vi "Get DIP State.vi"(8 "error in (no error)":errorcluster) -> (0 "error out":errorcluster, 3 "DIP State":u32)   [LabVIEW 2016]
uses:
  Refname/Sensors.ctl
  Refname/Refname to String (Sensors).vi
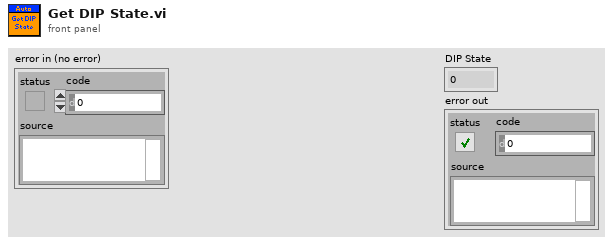
[diagram p1: front panel]
types:
  T1 = typedef "Sensors.ctl" = enum16{"DIP 1", "DIP 2", "DIP 3", "DIP 4", "IMU", "HuskieBoard"}
  T2 = typedef "WPI_SwitchDevRef.ctl" = cluster{"DevStatus":errorcluster, "DIO Channel":T3, "CntIndex":T4, "Normally Closed":bool}
  T3 = typedef "FPGA_DIOChannel.ctl" = enum8{"DIO 0", "DIO 1", "DIO 2", "DIO 3", "DIO 4", "DIO 5", "DIO 6", "DIO 7", "DIO 8", "DIO 9", "DIO MXP 0", "DIO MXP 1", "DIO MXP 2", "DIO MXP 3", "DIO MXP 4", "DIO MXP 5", "DIO MXP 6", "DIO MXP 7", "DIO MXP 8", "DIO MXP 9", "DIO MXP 10", "DIO MXP 11", "DIO MXP 12", "DIO MXP 13", "DIO MXP 14", "DIO MXP 15", "SPI Port CS1", "SPI Port CS2", "SPI Port CS3", "SPI Port MISO", "SPI Port MOSI", "Invalid"}
  T4 = typedef "FPGA_CounterCtrSystemIndex.ctl" = enum8{"Ctr 0", "Ctr 1", "Ctr 2", "Ctr 3", "Ctr 4", "Ctr 5", "Ctr 6", "Ctr 7", "Invalid"}
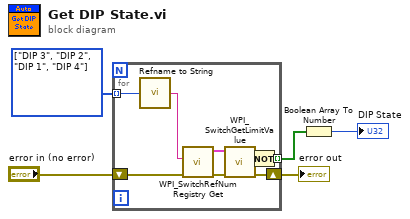
[diagram p0: block diagram]
diagram:
  w5 = T1[] [enum."DIP 3", enum."DIP 2", enum."DIP 1", enum."DIP 4"] items=["DIP 1", "DIP 2", "DIP 3", "DIP 4", "IMU", "HuskieBoard"]
  n1 = for {
    tunnel: w5 -> [w12] mode=indexing
    shift-right: [w9] -> w2
    shift-left: "error in (no error)" -> [w11]
    tunnel: [w6] -> w1 mode=indexing
    n2 = call-poly "Refname to String.vi"("Enum"=w12) -> ("String"=w13:string)
    n3 = call <vilib>:"WPI_SwitchRefNum Registry Get.vi"("error in (no error)"=w11, "refnum name"=w13) -> ("error out"=w10:errorcluster, "SwitchDevRef"=w8:T2)  [unwired: 8 in]
    n4 = call <vilib>:"WPI_SwitchGetLimitValue.vi"("error in (no error)"=w10, "SwitchDevRef"=w8) -> ("error out"=w9:errorcluster, "Switch Pressed"=w7:bool)  [unwired: 7 in, 1 out]
    n5 = Not(x=w7) -> (.not. x?=w6:bool)
  }
  "error out" <- w2
  n6 = Boolean Array To Number(Boolean array=w1) -> (number=→"DIP State":u32)
